vi "Loop Operation.vi"(8 "error in (no error)":errorcluster, 11 "BLE context in":refnum<class "BLE context.lvclass">) -> (0 "error out":errorcluster, 2 "BLE Message out":refnum<class "BLE Message.lvclass">, 3 "BLE context out":refnum<class "BLE context.lvclass">)   [LabVIEW 2015, in "BLE context.lvclass"]
uses:
  BLE context.lvclass
  BLE Message/BLE Message.lvclass
  BLE context.lvclass/BLE context.ctl
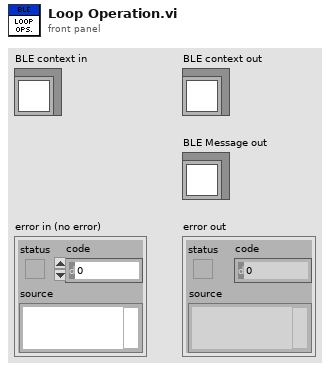
[diagram p1: front panel]
types:
  T1 = typedef "RefsBox.ctl" = cluster{"Heart Rate Plot ref":refnum<vi>, "Accelerometers":refnum<vi>, "Main VI":refnum<vi>}
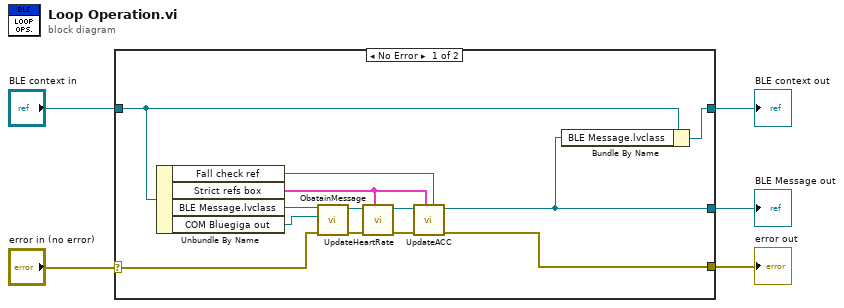
[diagram p0: block diagram]
diagram:
  n1 = case shown="No Error" "error in (no error)" {
    selector: "error in (no error)" -> [w16 w20]
    tunnel: [w7 w20] -> w4
    tunnel: [w13 w19] -> w2
    tunnel: "BLE context in" -> [w12 w19]
    tunnel: [w8 _] -> w1
    frame No Error {
      n2 = Unbundle By Name(w12) -> ("Fall check ref"=w6:refnum<k24>, "Strict refs box"=w9:T1, "BLE Message.lvclass"=w18:refnum<class "BLE Message.lvclass">, "COM Bluegiga out"=w17:refnum<visa-resource-name>)
      n3 = call "ObatainMessage.vi"("error in (no error)"=w16, "COM Bluegiga in"=w17, "BLE Message in"=w18) -> ("error out"=w14:errorcluster, "BLE Message out"=w15:refnum<class "BLE Message.lvclass">)  [unwired: 7 in]
      n4 = call "UpdateHeartRate.vi"("Strict refs box"=w9, "error in (no error)"=w14, "BLE Message in"=w15) -> ("error out"=w10:errorcluster, "BLE Message out"=w11:refnum<class "BLE Message.lvclass">)  [unwired: 7 in]
      n5 = call "UpdateACC.vi"("Fall check ref"=w6, "Strict refs box"=w9, "error in (no error)"=w10, "BLE Message in"=w11) -> ("error out"=w7:errorcluster, "BLE Message out"=w8:refnum<class "BLE Message.lvclass">)  [unwired: 6 in]
      n6 = Bundle By Name(cluster=w12, "BLE Message.lvclass"=w8) -> (w13:refnum<class "BLE context.lvclass">)
    }
    frame Error {
    }
  }
  "error out" <- w4
  "BLE context out" <- w2
  "BLE Message out" <- w1
